vi "SEND_CONFIG.vi"(8 "error in":errorcluster caption="에러 출력", 11 "TCP_In":refnum<k5>) -> (0 "error out":errorcluster caption="에러 출력", 3 "TCP_Out":refnum<k5>)   [LabVIEW 2019]
uses:
  Type/Type_TCP_Cmd.ctl
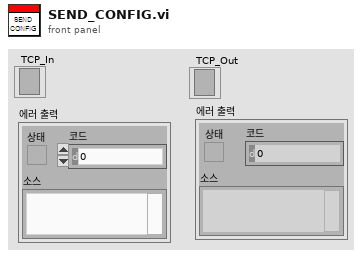
[diagram p1: front panel]
types:
  T1 = typedef "Type_TCP_Cmd.ctl" = enum16{"None", "Data", "Config", "Active"}
  T2 = cluster{"Init_Onset_Load":sgl, "Param":cluster{"Clt_Param_L":cluster{"기준값":sgl, "검출값":sgl, "Onset_Min":sgl, "Onset_Max":sgl, "Peak_Min":sgl, "Peak_Max":sgl, "Base":i32}, "Clt_Param_R":cluster{"기준값":sgl, "검출값":sgl, "Onset_Min":sgl, "Onset_Max":sgl, "Peak_Min":sgl, "Peak_Max":sgl, "Base":i32}}, "MinPos":i32, "MaxPos":i32, "Init_Vel_UP":i32, "Init_Accel":u32, "Test_Vel":i32, "Test_Acc":u32, "Init_Vel_DOWN":i32, "Load_Warning":sgl, "Load_Alarm":sgl}
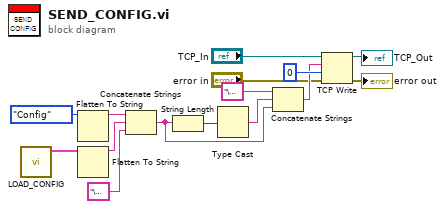
[diagram p0: block diagram]
diagram:
  n1 = call "LOAD_CONFIG.vi"() -> ("Param"=w1:T2)  [unwired: 10 in, 1 out]
  n2 = Flatten To String(anything=Type_TCP_Cmd."Config") -> (data string=w9:string)  [unwired: 3 in, 2 out]
  n3 = Flatten To String(anything=w1) -> (data string=w10:string)  [unwired: 3 in, 2 out]
  n4 = Concatenate Strings(w9, w10, "\u0003" ("문자열")) -> (w14:string)
  n5 = String Length(string=w14) -> (length=w11:i32)
  n6 = Type Cast(x=w11) -> (*(type *) &x=w12:string)  [unwired: 1 in]
  n7 = Concatenate Strings("\u0002" ("문자열"), w12, w14) -> (w7:string)
  n8 = TCP Write(connection ID="TCP_In", data in=w7, error in (no error)="error in", 9:0 ("타임아웃 ms (25000)")) -> (connection ID out=→"TCP_Out":refnum<k5>, error out=→"error out":errorcluster)  [unwired: 1 out]
